vi "Control WavePond.vi"(6 "working directory":path=path "", 8 "Error In":errorcluster, 9 "Parameter":string, 10 "Command":T1) -> (0 "Error Out":errorcluster, 2 "Return Message":string, 3 "standard output":string)   [LabVIEW 2014, in "Wavepond.lvclass"]
uses:
  Wavepond.lvclass
  Wavepond Commands.ctl
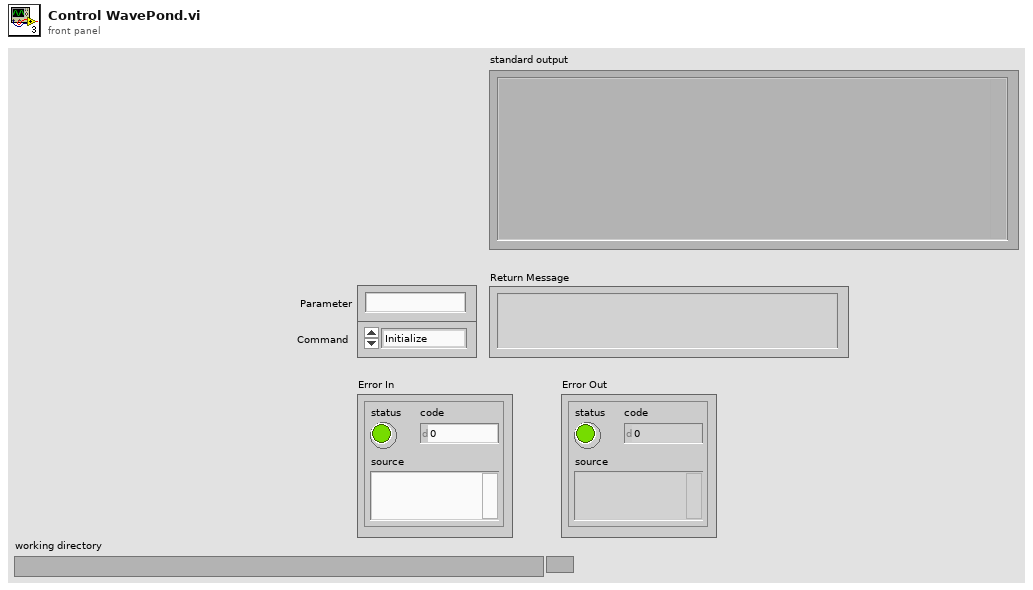
[diagram p1: front panel]
types:
  T1 = typedef "Wavepond Commands.ctl" = enum16{"Initialize", "SetFrequency", "SetAtten", "WriteData", "EnableSweep", "SetLoopCnt", "SetClkDiv", "SelExtTrig", "SoftTrig", "En_SqWave"}
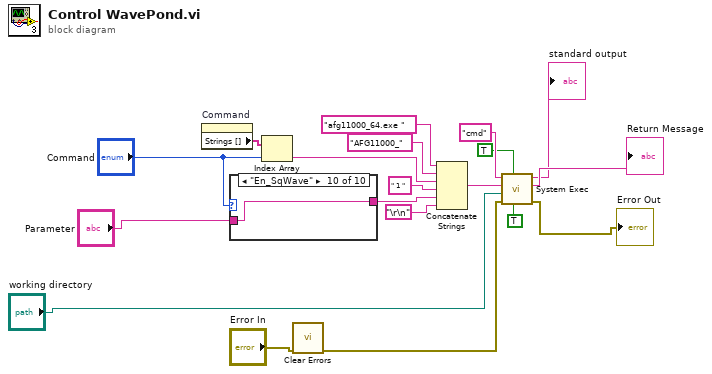
[diagram p0: block diagram]
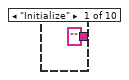
[diagram p2: hidden frame]
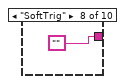
[diagram p9: hidden frame]
diagram:
  n1 = property on="Command" class="Enum (strict)"() -> ("Strings []"=w11:string[])  [unwired: 2 in, 2 out]
  n2 = case shown="\"En_SqWave\"" "Command" {
    tunnel: ["" ("Parameter") w21 w22 w23 w24 w25 w26 "" w28 w29] -> w13
    tunnel: "Parameter" -> [_ w21 w22 w23 w24 w25 w26 _ w28 w29]
    frame "Initialize" {
    }
    frame "SetFrequency" {
    }
    frame "SetAtten" {
    }
    frame "WriteData" {
    }
    frame "EnableSweep" {
    }
    frame "SetLoopCnt" {
    }
    frame "SetClkDiv" {
    }
    frame "SoftTrig" {
    }
    frame "SelExtTrig" {
    }
    frame "En_SqWave" {
    }
  }
  n3 = Index Array(array=w11, index="Command") -> (element=w10:string)
  n4 = call <vilib>:"Clear Errors.vi"("error in (no error)"="Error In") -> ("error out"=w3:errorcluster)  [unwired: 5 in, 1 out]
  n5 = Concatenate Strings("afg11000_64.exe " ("string"), "AFG11000_" ("string"), w10, " 1 " ("string"), w13, "\r\n") -> (w12:string)
  n6 = call <vilib>:"System Exec.vi"("run minimized? (F)"=TRUE, "wait until completion? (T)"=TRUE, "error in (no error)"=w3, "working directory"="working directory", "standard input"=w12, "command line"="cmd") -> ("error out"=→"Error Out":errorcluster, "standard error"=→"Return Message":string, "standard output"=→"standard output":string)  [unwired: 2 in, 1 out]
